vi "Modified Measuring Y verses V.vi"() -> ()   [LabVIEW 2020]
uses:
  <vilib>/DAQmx/write.llb/DAQmx Write (Analog Wfm 1Chan NSamp).vi
  <vilib>/DAQmx/create/channels.llb/DAQmx Create Channel (AO-Voltage-Basic).vi
  <vilib>/Utility/file.llb/Read Delimited Spreadsheet (DBL).vi
  <vilib>/DAQmx/configure/timing.llb/DAQmx Timing (Sample Clock).vi
  <vilib>/DAQmx/miscellaneous.llb/DAQmx Fill In Error Info.vi
  <vilib>/DAQmx/create/channels.llb/DAQmx Create Channel (CO-Pulse Generation-Frequency).vi
  <vilib>/DAQmx/configure/timing.llb/DAQmx Timing (Implicit).vi
  <resource>/objmgr/daqmx.rc
panel:
  out "actual frequency":dbl
  in  "stop":bool
  out "Signal input to voice coil (blue)":dbl[](graph)=[-0.285]
  in  "file path (dialog if empty) 2":path=path "C:/Users/htm22/Downloads/Voltage_positions_500.txt"
  out "# Samples written per channel":u32
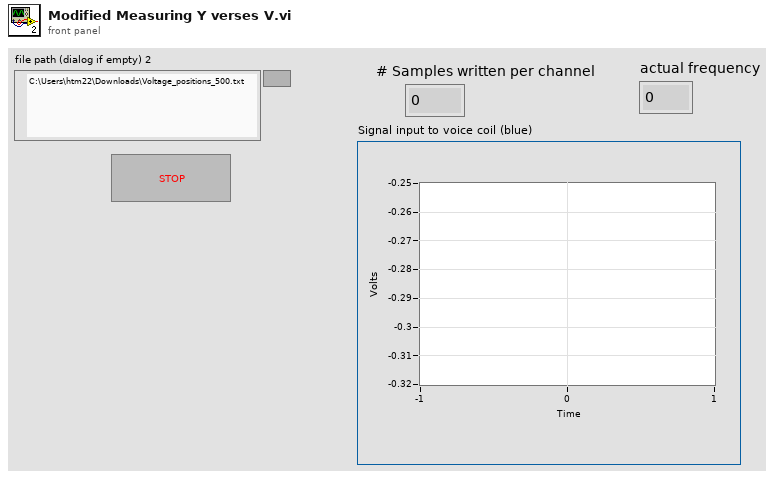
[diagram p1: front panel]
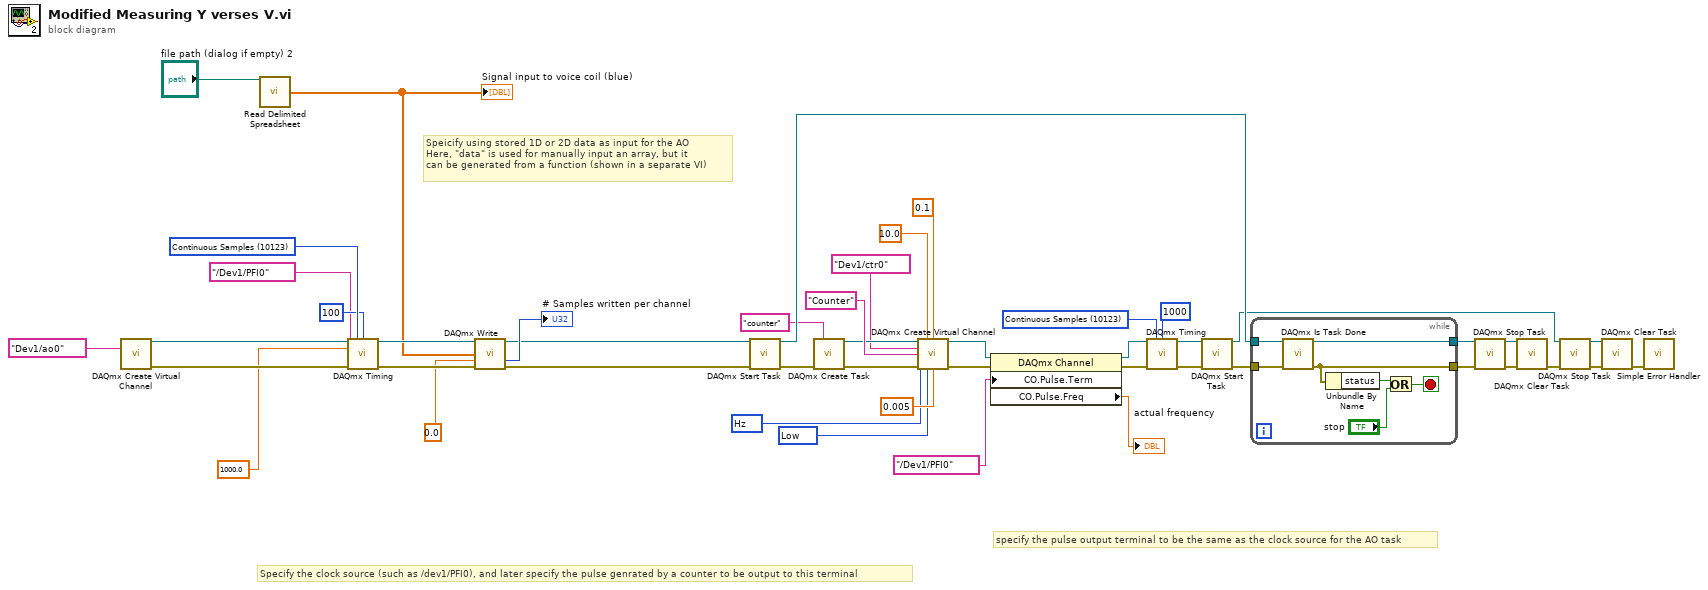
[diagram p0: block diagram]
diagram:
  w6 = 10214 items=["High"=10192, "Low"=10214] ("idle state")
  w7 = 10373 items=["Hz"=10373] ("units")
  w38 = 10123 items=["Finite Samples"=10178, "Continuous Samples"=10123, "Hardware Timed Single Point"=12522] ("sample mode")
  w45 = 10123 items=["Finite Samples"=10178, "Continuous Samples"=10123, "Hardware Timed Single Point"=12522] ("sample mode")
  # "specify the pulse output terminal to be the same as the clock source for the AO task"
  # "Speicify using stored 1D or 2D data as input for the AO\nHere, \"data\" is used for manually input an array, but it\ncan be generated from a function (shown in a separate VI)"
  # "Specify the clock source (such as /dev1/PFI0), and later specify the pulse genrated by a counter to be output to this terminal"
  n1 = call-poly <vilib>:"DAQmx Create Virtual Channel.vi"("physical channels"=tag "Dev1/ao0") -> ("task out"=w47:refnum<k21>, "error out"=w46:errorcluster)  [unwired: 13 in]
  n2 = call-poly <vilib>:"Read Delimited Spreadsheet.vi"("file path (dialog if empty)"="file path (dialog if empty) 2") -> ("first row"=w4:dbl[])  [unwired: 9 in, 5 out]
  "Signal input to voice coil (blue)" <- w4
  n3 = call-poly <vilib>:"DAQmx Timing.vi"("task/channels in"=w47, "sample mode"=w45, "samples per channel"=100, "rate"=1000.0, "source"=tag "/Dev1/PFI0", "error in"=w46) -> ("task out"=w41:refnum<k21>, "error out"=w44:errorcluster)  [unwired: 8 in]
  n4 = call-poly <vilib>:"DAQmx Write.vi"("task/channels in"=w41, "data"=w4, "timeout"=0.0, "error in"=w44) -> ("task out"=w15:refnum<k21>, "number of samples written per channel"=→"# Samples written per channel":u32, "error out"=w14:errorcluster)  [unwired: 9 in]
  n5 = call <vilib>:"DAQmx Start Task.vi"("task/channels in"=w15, "error in"=w14) -> ("task out"=w39:refnum<k21>, "error out"=w17:errorcluster)  [unwired: 12 in]
  n6 = call <vilib>:"DAQmx Create Task.vi"("new task name"="counter", "error in"=w17) -> ("task out"=w34:refnum<k21>, "error out"=w32:errorcluster)  [unwired: 12 in]
  n7 = call-poly <vilib>:"DAQmx Create Virtual Channel.vi"("task in"=w34, "frequency"=10.0 ("rate"), "duty cycle"=0.1, "counter"=tag "Dev1/ctr0", "name to assign"="Counter", "units"=w7, "error in"=w32, "idle state"=w6, "initial delay"=0.005) -> ("task out"=w31:refnum<k21>, "error out"=w30:errorcluster)  [unwired: 5 in]
  n8 = property class="DAQmx Channel"(reference=w31, error in=w30, "CO.Pulse.Term"=tag "/Dev1/PFI0") -> (reference out=w27:refnum<k21>, error out=w28:errorcluster, "CO.Pulse.Freq"=→"actual frequency":dbl)
  n9 = call-poly <vilib>:"DAQmx Timing.vi"("task/channels in"=w27, "sample mode"=w38, "samples per channel"=1000, "error in"=w28) -> ("task out"=w37:refnum<k21>, "error out"=w36:errorcluster)  [unwired: 10 in]
  n10 = call <vilib>:"DAQmx Start Task.vi"("task/channels in"=w37, "error in"=w36) -> ("task out"=w26:refnum<k21>, "error out"=w16:errorcluster)  [unwired: 12 in]
  n11 = while {
    tunnel: w39 -> [w54]
    tunnel: w16 -> [w53]
    tunnel: [w52] -> w22
    tunnel: [w51] -> w23
    stop <- w48 stop-if-true
    n12 = call <vilib>:"DAQmx Is Task Done.vi"("task/channels in"=w54, "error in"=w53) -> ("task out"=w52:refnum<k21>, "error out"=w51:errorcluster)  [unwired: 11 in, 1 out]
    n13 = Unbundle By Name(w51) -> ("status"=w50:bool)
    n14 = Or(x=w50, y="stop") -> (x .or. y?=w48:bool)
  }
  n15 = call <vilib>:"DAQmx Stop Task.vi"("task/channels in"=w22, "error in"=w23) -> ("task out"=w21:refnum<k21>, "error out"=w20:errorcluster)  [unwired: 12 in]
  n16 = call <vilib>:"DAQmx Clear Task.vi"("task in"=w21, "error in"=w20) -> ("error out"=w19:errorcluster)  [unwired: 13 in]
  n17 = call <vilib>:"DAQmx Stop Task.vi"("task/channels in"=w26, "error in"=w19) -> ("task out"=w24:refnum<k21>, "error out"=w25:errorcluster)  [unwired: 12 in]
  n18 = call <vilib>:"DAQmx Clear Task.vi"("task in"=w24, "error in"=w25) -> ("error out"=w18:errorcluster)  [unwired: 13 in]
  n19 = call <vilib>:"Simple Error Handler.vi"("error in (no error)"=w18) -> ()  [unwired: 4 in, 5 out]
